vi "Get_CPU_Model_Name.vi"() -> (3 "CPU Model":string)   [LabVIEW 2020]
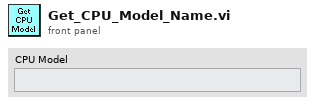
[diagram p1: front panel]
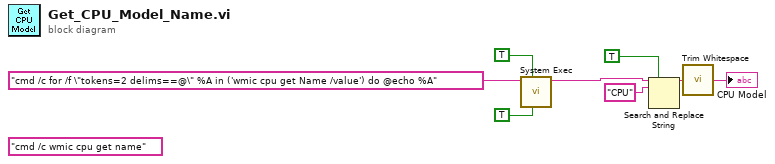
[diagram p0: block diagram]
diagram:
  (unwired) "cmd /c wmic cpu get name" ("command line")
  n1 = call <vilib>:"System Exec.vi"("run minimized? (F)"=TRUE, "wait until completion? (T)"=TRUE, "command line"="cmd /c for /f \"tokens=2 delims==@\" %A in ('wmic cpu get Name /value') do @echo %A") -> ("standard output"=w4:string)  [unwired: 5 in, 3 out]
  n2 = Search and Replace String(replace all?=TRUE ("replace all? (F)"), input string=w4, search string="CPU") -> (result string=w5:string)  [unwired: 5 in, 3 out]
  n3 = call <vilib>:"Trim Whitespace.vi"("string"=w5) -> ("trimmed string"=→"CPU Model":string)  [unwired: 1 in]
